vi "newTestStandCustomType.vi"(0 "Engine Reference":refnum<k7>, 5 "Sequence File Ref":refnum<k7>, 11 "error in":errorcluster) -> (4 "Engine Reference (out)":refnum<k7>, 6 "Sequence File (out)":refnum<k7>, 15 "error out":errorcluster)   [LabVIEW 2009]
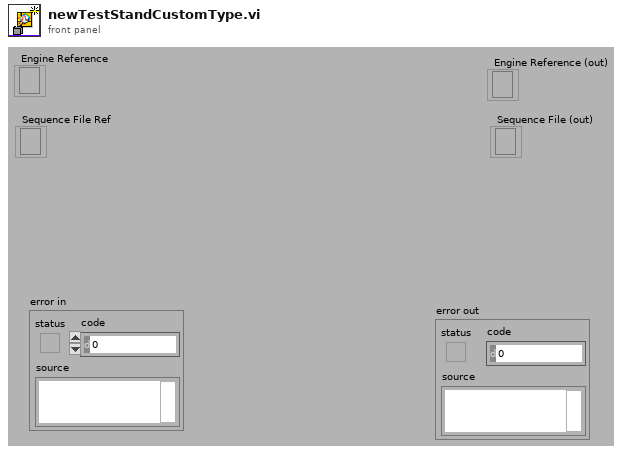
[diagram p1: front panel]
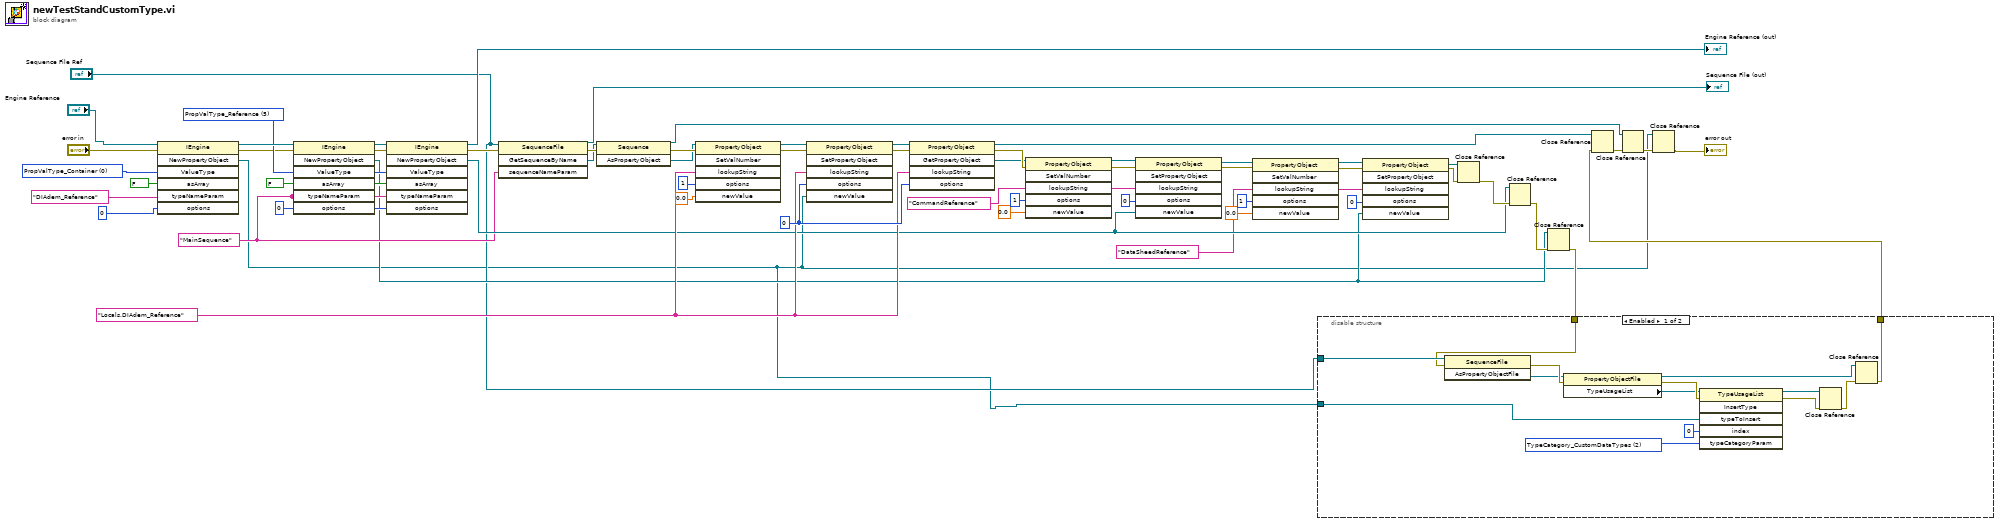
[diagram p0: block diagram]
diagram:
  w53 = "Locals.DIAdem_Reference" ("Variable Name")
  w22 = "DataSheedReference" ("lookupString")
  w32 = "CommandReference" ("lookupString")
  w26 = FALSE ("asArray")
  w24 = 0 ("options")
  w27 = 5 items=["PropValType_Container", "PropValType_String", "PropValType_Boolean", "PropValType_Number", "PropValType_NamedType", "PropValType_Reference", "PropValType_Array"] ("ValueType")
  w56 = 0 items=["PropValType_Container", "PropValType_String", "PropValType_Boolean", "PropValType_Number", "PropValType_NamedType", "PropValType_Reference", "PropValType_Array"] ("ValueType")
  w54 = 0 ("options")
  w25 = "MainSequence" ("sequenceNameParam")
  n1 = invoke class="IEngine" method="NewPropertyObject"(reference="Engine Reference", error in="error in", "ValueType"=w56, "asArray"=FALSE, "typeNameParam"="DIAdem_Reference", "options"=0) -> (reference out=w28:refnum<k7>, error out=w11:errorcluster, "NewPropertyObject"=w1:refnum<k7>)  [unwired: 1 in, 4 out]
  n2 = invoke class="IEngine" method="NewPropertyObject"(reference=w28, error in=w11, "ValueType"=w27, "asArray"=w26, "typeNameParam"=w25, "options"=w24) -> (reference out=w30:refnum<k7>, error out=w29:errorcluster, "NewPropertyObject"=w5:refnum<k7>)  [unwired: 1 in, 4 out]
  n3 = invoke class="IEngine" method="NewPropertyObject"(reference=w30, error in=w29, "ValueType"=w27, "asArray"=w26, "typeNameParam"=w25, "options"=w24) -> (reference out=→"Engine Reference (out)":refnum<k7>, error out=w39:errorcluster, "NewPropertyObject"=w37:refnum<k7>)  [unwired: 1 in, 4 out]
  n4 = invoke class="SequenceFile" method="GetSequenceByName"(reference="Sequence File Ref", error in=w39, "sequenceNameParam"=w25) -> (reference out=→"Sequence File (out)":refnum<k7>, error out=w47:errorcluster, "GetSequenceByName"=w7:refnum<k7>)  [unwired: 1 in, 1 out]
  n5 = invoke class="Sequence" method="AsPropertyObject"(reference=w7, error in=w47) -> (reference out=w48:refnum<k7>, error out=w45:errorcluster, "AsPropertyObject"=w2:refnum<k7>)  [unwired: 1 in]
  n6 = invoke class="PropertyObject" method="SetValNumber"(reference=w2, error in=w45, "lookupString"=w53, "options"=1, "newValue"=0.0) -> (reference out=w55:refnum<k7>, error out=w50:errorcluster)  [unwired: 1 in, 4 out]
  n7 = invoke class="PropertyObject" method="SetPropertyObject"(reference=w55, error in=w50, "lookupString"=w53, "options"=w54, "newValue"=w1) -> (reference out=w12:refnum<k7>, error out=w51:errorcluster)  [unwired: 1 in, 4 out]
  n8 = invoke class="PropertyObject" method="GetPropertyObject"(reference=w12, error in=w51, "lookupString"=w53, "options"=w54) -> (reference out=w52:refnum<k7>, error out=w42:errorcluster, "GetPropertyObject"=w3:refnum<k7>)  [unwired: 1 in, 2 out]
  n9 = invoke class="PropertyObject" method="SetValNumber"(reference=w3, error in=w42, "lookupString"=w32, "options"=1, "newValue"=0.0) -> (reference out=w34:refnum<k7>, error out=w33:errorcluster)  [unwired: 1 in, 4 out]
  n10 = invoke class="PropertyObject" method="SetPropertyObject"(reference=w34, error in=w33, "lookupString"=w32, "options"=0, "newValue"=w37) -> (reference out=w15:refnum<k7>, error out=w14:errorcluster)  [unwired: 1 in, 4 out]
  n11 = invoke class="PropertyObject" method="SetValNumber"(reference=w15, error in=w14, "lookupString"=w22, "options"=1, "newValue"=0.0) -> (reference out=w20:refnum<k7>, error out=w21:errorcluster)  [unwired: 1 in, 4 out]
  n12 = invoke class="PropertyObject" method="SetPropertyObject"(reference=w20, error in=w21, "lookupString"=w22, "options"=0, "newValue"=w5) -> (reference out=w16:refnum<k7>, error out=w17:errorcluster)  [unwired: 1 in, 4 out]
  n13 = Close Reference(reference=w16, error in (no error)=w17) -> (error out=w40:errorcluster)
  n14 = Close Reference(reference=w37, error in (no error)=w40) -> (error out=w13:errorcluster)
  n15 = Close Reference(reference=w5, error in (no error)=w13) -> (error out=w9:errorcluster)
  n16 = disable-structure shown="Enabled" {
    disable-tunnel: "Sequence File Ref" -> [w70 _]
    disable-tunnel: w9 -> [w68 w75]
    disable-tunnel: [w67 w75] -> w8
    disable-tunnel: w1 -> [w63 _]
    frame #0 {
      w69 = 2 items=["TypeCategory_None", "TypeCategory_StepTypes", "TypeCategory_CustomDataTypes", "TypeCategory_BuiltinDataTypes"] ("typeCategoryParam")
      n17 = invoke class="SequenceFile" method="AsPropertyObjectFile"(reference=w70, error in=w68) -> (error out=w73:errorcluster, "AsPropertyObjectFile"=w65:refnum<k7>)  [unwired: 1 in, 1 out]
      n18 = property class="PropertyObjectFile"(reference=w65, error in=w73) -> (reference out=w71:refnum<k7>, error out=w74:errorcluster, "TypeUsageList"=w61:refnum<k7>)
      n19 = invoke class="TypeUsageList" method="InsertType"(reference=w61, error in=w74, "typeToInsert"=w63, "index"=0, "typeCategoryParam"=w69) -> (reference out=w64:refnum<k7>, error out=w62:errorcluster)  [unwired: 1 in, 4 out]
      n20 = Close Reference(reference=w64, error in (no error)=w62) -> (error out=w72:errorcluster)
      n21 = Close Reference(reference=w71, error in (no error)=w72) -> (error out=w67:errorcluster)
    }
    frame #1 {
    }
  }
  n22 = Close Reference(reference=w52, error in (no error)=w8) -> (error out=w41:errorcluster)
  n23 = Close Reference(reference=w48, error in (no error)=w41) -> (error out=w60:errorcluster)
  n24 = Close Reference(reference=w1, error in (no error)=w60) -> (error out=→"error out":errorcluster)
